vi "Read Input Modules at Indexes.vi"(5 "Indexes":i32[](array[numeric]), 7 "R/W Case":T12, 8 "error in (no error)":errorcluster, 10 "Async in in":T13, 11 "RSI Modules in in":T1[](array[typedef]) {"Module Config Data"."Config Block Data Refs"."Data Reference" format="%.0x"; "CDOutput Data"."BD Refs"."Data Reference" format="%.0x"; "CDInput Data"."BD Refs"."Data Reference" format="%.0x"; "VS ref" format="%.0x"}) -> (0 "error out":errorcluster, 2 "Async in out":T13, 3 "RSI Modules in out":T1[](array[typedef]) {"Module Config Data"."Config Block Data Refs"."Data Reference" format="%.0x"; "CDOutput Data"."BD Refs"."Data Reference" format="%.0x"; "CDInput Data"."BD Refs"."Data Reference" format="%.0x"; "VS ref" format="%.0x"})   [LabVIEW 2020, in "SEECD Engine.lvlib"]
uses:
  SEECD Engine.lvlib
  Type Defs/Async Command.ctl
  Type Defs/Async State.ctl
  Type Defs/Async Status.ctl
  Type Defs/Async Data.ctl
  <vilib>/NI VeriStand/Custom Device API/Custom Device Item Ref.ctl
  <vilib>/NI VeriStand/Custom Device API/Custom Device API.lvlib
  <vilib>/NI VeriStand/Custom Device API/Data Reference.ctl
  <vilib>/NI VeriStand/Custom Device API/Block Data Reference.ctl
  Type Defs/Input Data.ctl
  Type Defs/Output Data.ctl
  Includes/Modules.lvlibp/RSI Module/Channel Type.ctl
  Includes/Modules.lvlibp/RSI Module/RSI Module.lvclass
  Includes/Modules.lvlibp/RSI Module/Module Models.ctl
  Type Defs/Module Config Data.ctl
  Type Defs/Mixed IO.ctl
  Type Defs/Open Module IOVs.ctl
  Type Defs/RSI Module Data.ctl
  Type Defs/RW Case.ctl
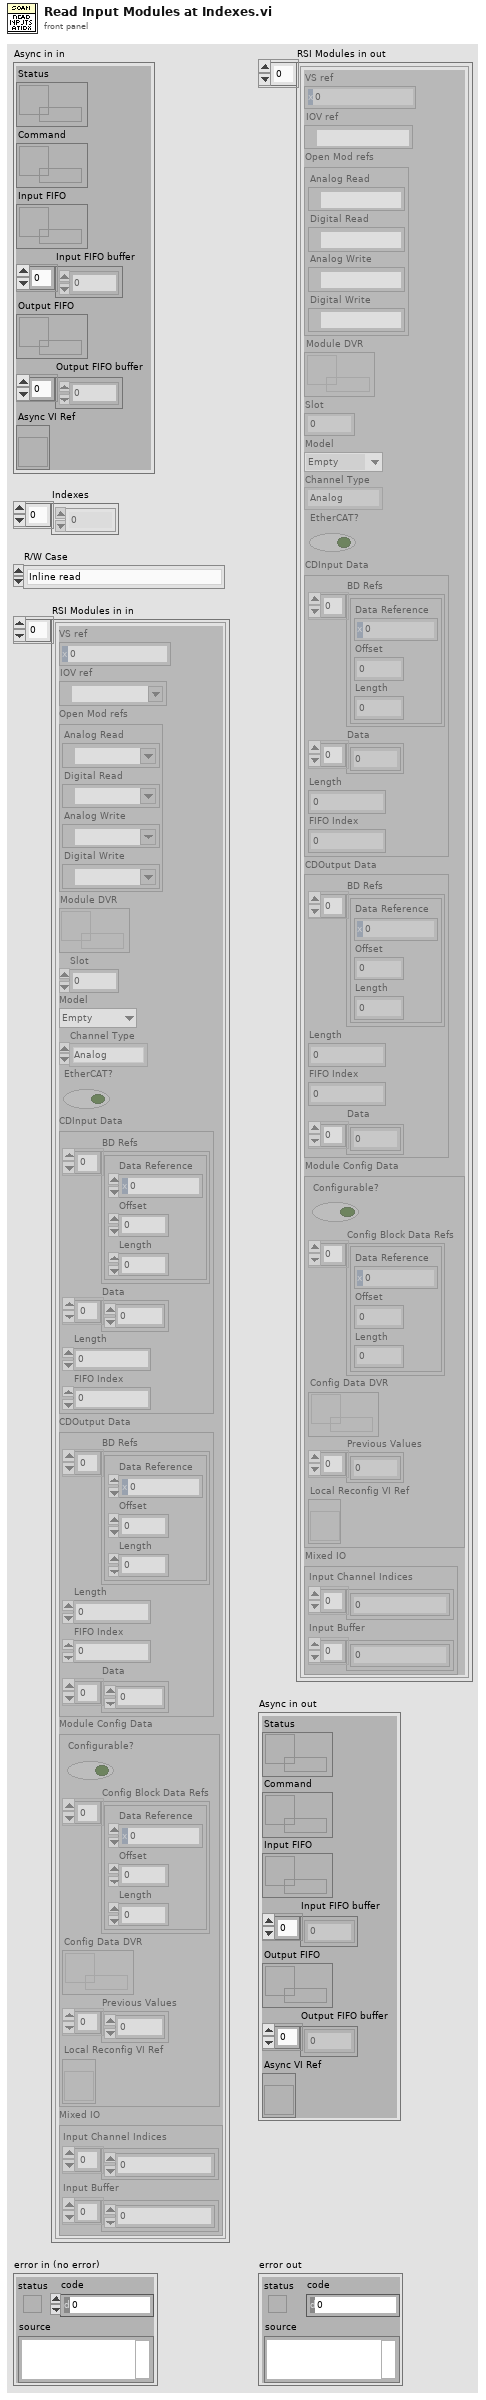
[diagram p1: front panel]
types:
  T1 = typedef "SEECD Engine.lvlib/RSI Module Data.ctl" = cluster{"VS ref":T2, "IOV ref":refnum<k21>, "Open Mod refs":T3, "Module DVR":refnum<data-value>, "Slot":u32, "Model":T4, "Channel Type":T5, "EtherCAT?":bool, "CDInput Data":T6, "CDOutput Data":T9, "Module Config Data":T10, "Mixed IO":T11}
  T2 = typedef "Custom Device API.lvlib/Custom Device Item Ref.ctl" = u64
  T3 = typedef "SEECD Engine.lvlib/Open Module IOVs.ctl" = cluster{"Analog Read":refnum<k21>, "Digital Read":refnum<k21>, "Analog Write":refnum<k21>, "Digital Write":refnum<k21>}
  T4 = typedef "Modules.lvlibp/RSI Module.lvclass/Module Models.ctl" = enum16{"Empty", "NI 9201", "NI 9203", "NI 9205", "NI 9206", "NI 9207", "NI 9208", "NI 9209", "NI 9210", "NI 9211", "NI 9212", "NI 9213", "NI 9214", "NI 9215", "NI 9216", "NI 9217", "NI 9219", "NI 9220", "NI 9221", "NI 9222", "NI 9223", "NI 9224", "NI 9225", "NI 9226", "NI 9227", "NI 9228", "NI 9229", "NI 9233", "NI 9234", "NI 9235", "NI 9236", "NI 9237", "NI 9239", "NI 9242", "NI 9244", "NI 9253", "NI 9263", "NI 9264", "NI 9265", "NI 9266", "NI 9269", "NI 9344", "NI 9350", "NI 9375", "NI 9401", "NI 9402", "NI 9403", "NI 9411", "NI 9421", "NI 9422", "NI 9423", "NI 9425", "NI 9426", "NI 9435", "NI 9436", "NI 9437", "NI 9472", "NI 9474", "NI 9475", "NI 9476", "NI 9477", "NI 9478", "NI 9481", "NI 9482", "NI 9485"}
  T5 = typedef "Modules.lvlibp/RSI Module.lvclass/Channel Type.ctl" = enum16{"Analog", "Digital"}
  T6 = typedef "SEECD Engine.lvlib/Input Data.ctl" = cluster{"BD Refs":T7[], "Data":dbl[], "Length":i32, "FIFO Index":i32}
  T7 = typedef "Custom Device API.lvlib/Block Data Reference.ctl" = cluster{"Data Reference":T8, "Offset":u64, "Length":u64}
  T8 = typedef "Custom Device API.lvlib/Data Reference.ctl" = i32
  T9 = typedef "SEECD Engine.lvlib/Output Data.ctl" = cluster{"BD Refs":T7[], "Length":i32, "FIFO Index":i32, "Data":dbl[]}
  T10 = typedef "SEECD Engine.lvlib/Module Config Data.ctl" = cluster{"Configurable?":bool, "Config Block Data Refs":T7[], "Config Data DVR":refnum<data-value>, "Previous Values":dbl[], "Local Reconfig VI Ref":refnum<vi>}
  T11 = typedef "SEECD Engine.lvlib/Mixed IO.ctl" = cluster{"Input Channel Indices":i32[], "Input Buffer":dbl[]}
  T12 = typedef "SEECD Engine.lvlib/RW Case.ctl" = enum16{"Inline read", "Inline write", "Async - Inline loop read", "Async - Inline loop write", "Async loop (read/write)"}
  T13 = typedef "SEECD Engine.lvlib/Async Data.ctl" = cluster{"Status":refnum<queue>, "Command":refnum<queue>, "Input FIFO":refnum<k33>, "Input FIFO buffer":dbl[], "Output FIFO":refnum<k33>, "Output FIFO buffer":dbl[], "Async VI Ref":refnum<vi>}
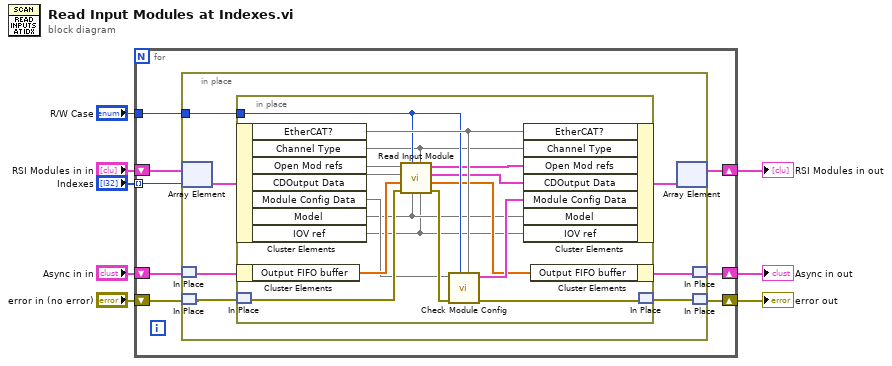
[diagram p0: block diagram]
diagram:
  n1 = for {
    shift-right: [w10] -> w3
    shift-left: "error in (no error)" -> [w11]
    shift-right: [w15] -> w1
    shift-left: "RSI Modules in in" -> [w16]
    tunnel: "R/W Case" -> [w14]
    shift-right: [w12] -> w4
    shift-left: "Async in in" -> [w13]
    tunnel: "Indexes" -> [w9] mode=indexing
    n2 = in-place {
      in-place-border: w14 -> [w21]
      n3 = in-place-array #1(w16, w9) -> (w23:T1)
      n4 = in-place-match #2(w13) -> (w20:T13)
      n5 = in-place-match #3(w11) -> (w18:errorcluster)
      n6 = in-place {
        in-place-border: w21 -> [w30]
        n7 = in-place-cluster #4(w23) -> ("EtherCAT?"=w31, "Channel Type"=w29, "Open Mod refs"=w37, "CDOutput Data"=w39, "Module Config Data"=w32, "Model"=w25, "IOV ref"=w24)
        n8 = in-place-cluster #5(w20) -> ("Output FIFO buffer"=w38:dbl[])
        n9 = in-place-match #6(w18) -> (w36:errorcluster)
        n10 = call "Read Input Module.vi"("IOV ref"=w24, "Channel Type"=w29, "Model"=w25, "R/W Case"=w30, "error in (no error)"=w36, "Output FIFO buffer in"=w38, "Output Data in"=w39, "IOV ref in"=w37) -> ("error out"=w33:errorcluster, "Output FIFO buffer out"=w26:dbl[], "Output Data out"=w27:T9, "IOV ref out"=w28:T3)
        n11 = call "Check Module Config.vi"("EtherCAT?"=w31, "R/W Case"=w30, "error in (no error)"=w33, "Module Config Data in"=w32) -> ("error out"=w35:errorcluster, "Module Config Data out"=w34:T10)  [unwired: 6 in]
        n12 = in-place-cluster #4("EtherCAT?"=w31, "Channel Type"=w29, "Open Mod refs"=w28, "CDOutput Data"=w27, "Module Config Data"=w34, "Model"=w25, "IOV ref"=w24) -> (w22:cluster{})
        n13 = in-place-cluster #5("Output FIFO buffer"=w26) -> (w19:T13)
        n14 = in-place-match #6(w35) -> (w17:errorcluster)
      }
      n15 = in-place-array #1(w22) -> (w15:T1[])  [unwired: 1 out]
      n16 = in-place-match #2(w19) -> (w12:T13)
      n17 = in-place-match #3(w17) -> (w10:errorcluster)
    }
  }
  "Async in out" <- w4
  "error out" <- w3
  "RSI Modules in out" <- w1
